vi "Data.vi"() -> ()   [LabVIEW 2020]
panel:
  out "Output":dbl[](array[numeric])
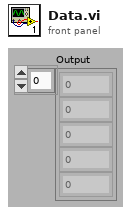
[diagram p1: front panel]
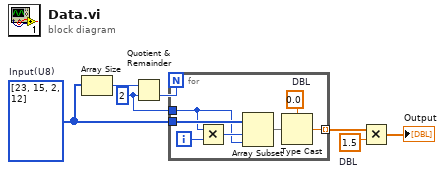
[diagram p0: block diagram]
diagram:
  w4 = 1.5  # DBL
  w5 = 2 ("y")
  w6 = i32[] [23, 15, 2, 12]  # Input(U8)
  n1 = Array Size(array=w6) -> (size(s)=w7:i32)
  n2 = Quotient & Remainder(x=w7, y=w5) -> (floor(x/y)=w1:i32)  [unwired: 1 out]
  n3 = for {
    N: w1 -> [_]
    tunnel: w6 -> [w14]
    tunnel: w5 -> [w11]
    tunnel: [w8] -> w3 mode=indexing
    i -> [w13]
    w9 = 0.0  # DBL
    n4 = Multiply(x=w11, y=w13) -> (x*y=w12:i32)
    n5 = Array Subset(array=w14, index=w12, length=w11) -> (w10:i32[])
    n6 = Type Cast(type=w9, x=w10) -> (*(type *) &x=w8:dbl)
  }
  n7 = Multiply(x=w3, y=w4) -> (x*y=→"Output":dbl[])
